vi "Map_Pos_sub_VI.vi"(8 "counter":i32, 9 "array":dbl[](array[numeric]), 10 "M1(t)/M2(f)":bool, 11 "Array":dbl[][](array[numeric])) -> (0 "counter out":i32, 3 "appended array":dbl[][](array[numeric]))   [LabVIEW 2018]
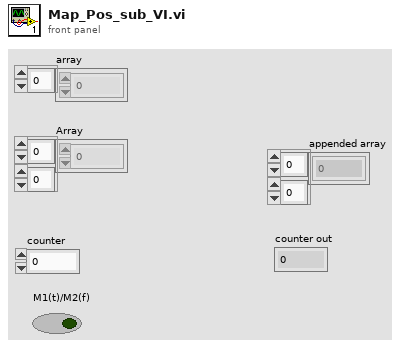
[diagram p1: front panel]
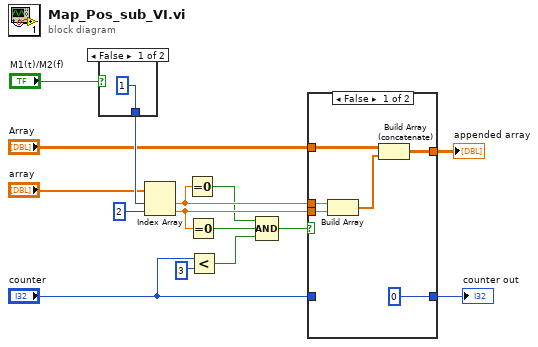
[diagram p0: block diagram]
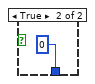
[diagram p2: hidden frame]
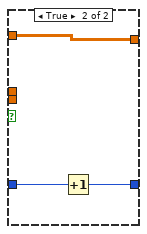
[diagram p3: hidden frame]
diagram:
  n1 = case shown="False" "M1(t)/M2(f)" {
    tunnel: [1 ("index") 0 ("index")] -> w15
    frame False {
    }
    frame True {
    }
  }
  n2 = Index Array(array="array", index #1=w15, index #2=2 ("index")) -> (element #1=w9:dbl, element #2=w10:dbl)
  n3 = Equal To 0?(x=w9) -> (x = 0?=w8:bool)
  n4 = Equal To 0?(x=w10) -> (x = 0?=w7:bool)
  n5 = Less?(x="counter", y=3) -> (x < y?=w2:bool)
  n6 = Compound Arithmetic op=AND(w8, w7, w2) -> (w6:bool)
  n7 = case shown="False" w6 {
    tunnel: "Array" -> [w23 w26]
    tunnel: [w22 w26] -> w12
    tunnel: w10 -> [w21 _]
    tunnel: w9 -> [w20 _]
    tunnel: "counter" -> [_ w25]
    tunnel: [0 w24] -> w5
    frame False {
      n8 = Build Array(w20, w21) -> (w19:dbl[])
      n9 = Build Array (concatenate)(w23, w19) -> (w22:dbl[][])
    }
    frame True {
      n10 = Increment(x=w25) -> (x+1=w24:i32)
    }
  }
  "appended array" <- w12
  "counter out" <- w5
